vi "Update limits.vi"(8 "error in (no error)":errorcluster, 10 "Experiment.lvclass in":refnum<class "Experiment.lvclass">, 11 "Control-Client in":refnum<class "Control-Client.lvclass">) -> (0 "error out":errorcluster, 3 "Control-Client out":refnum<class "Control-Client.lvclass">)   [LabVIEW 2018, in "Control-Client.lvclass"]
uses:
  Control-Client.lvclass
  Experiments/Experiment.lvclass
  Control-Client.lvclass/Control-Client.ctl
  Experiments/Experiment.lvclass/Experiment.ctl
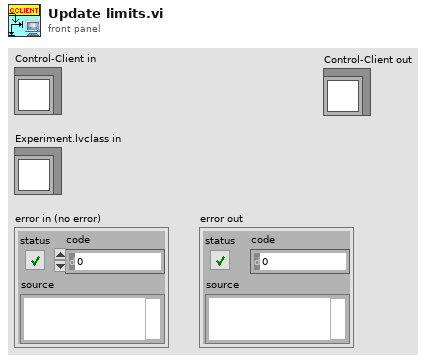
[diagram p1: front panel]
types:
  T1 = cluster{"From Time pix":i32, "To Time pix":i32, "From Wave pix":i32, "To Wave pix":i32}
  T2 = cluster{"waves slider":refnum<vi>, "times slider":refnum<vi>}
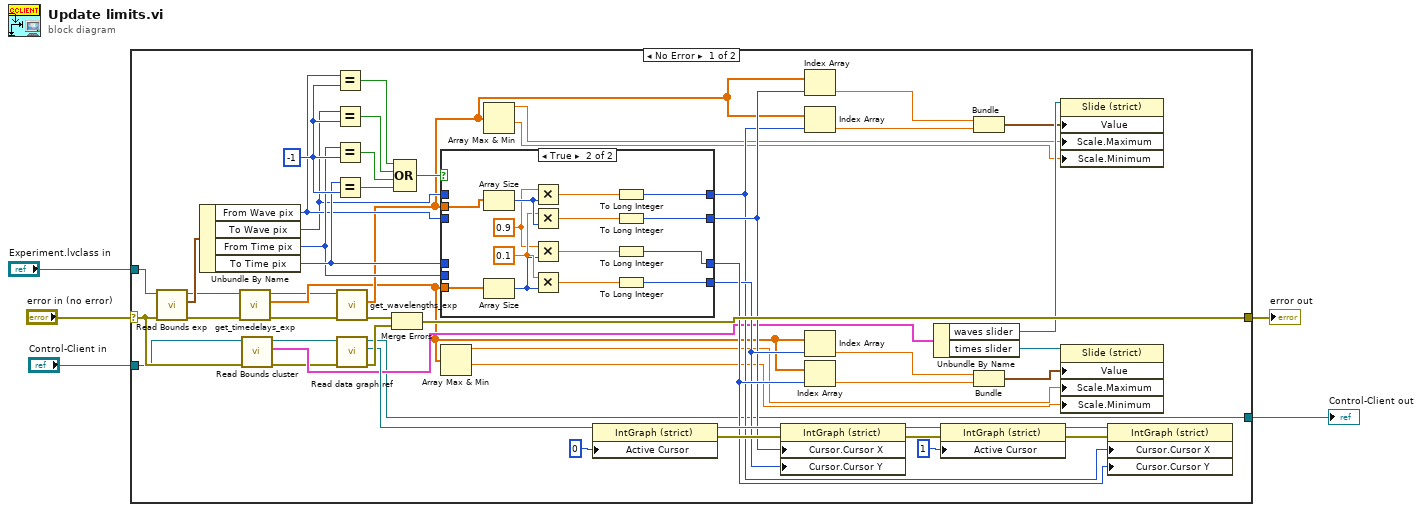
[diagram p0: block diagram]
diagram:
  n1 = case shown="No Error" "error in (no error)" {
    selector: "error in (no error)" -> [w43 w77]
    tunnel: "Experiment.lvclass in" -> [w57 _]
    tunnel: "Control-Client in" -> [w42 w76]
    tunnel: [w56 w77] -> w3
    tunnel: [w7 w76] -> w1
    frame No Error {
      w41 = -1 ("y")
      n2 = call "Read Bounds exp.vi"("error in (no error)"=w43, "Experiment in"=w57) -> ("error out"=w10:errorcluster, "Bounds pixels"=w44:T1, "Experiment out"=w12:refnum<class "Experiment.lvclass">)  [unwired: 7 in]
      n3 = Unbundle By Name(w44) -> ("From Wave pix"=w33:i32, "To Wave pix"=w29:i32, "From Time pix"=w34:i32, "To Time pix"=w35:i32)
      n4 = call "get_timedelays_exp.vi"("error in (no error)"=w10, "Experiment.lvclass in"=w12) -> ("error out"=w9:errorcluster, "timedelays"=w19:dbl[], "Experiment.lvclass out"=w11:refnum<class "Experiment.lvclass">)  [unwired: 7 in]
      n5 = call "Read Bounds cluster.vi"("error in (no error)"=w43, "Control-Client in"=w42) -> ("error out"=w6:errorcluster, "Bounds cluster"=w27:T2, "Control-Client out"=w8:refnum<class "Control-Client.lvclass">)  [unwired: 7 in]
      n6 = Equal?(x=w33, y=w41) -> (x = y?=w37:bool)
      n7 = Equal?(x=w29, y=w41) -> (x = y?=w38:bool)
      n8 = Equal?(x=w34, y=w41) -> (x = y?=w39:bool)
      n9 = Equal?(x=w35, y=w41) -> (x = y?=w40:bool)
      n10 = call "get_wavelengths_exp.vi"("error in (no error)"=w9, "Experiment.lvclass in"=w11) -> ("error out"=w45:errorcluster, "wavelengths"=w20:dbl[])  [unwired: 7 in, 1 out]
      n11 = call "Read data graph ref.vi"("error in (no error)"=w6, "Control-Client in"=w8) -> ("error out"=w55:errorcluster, "Exp data graph ref"=w54:refnum<vi>, "Control-Client out"=w7:refnum<class "Control-Client.lvclass">)  [unwired: 7 in]
      n12 = Merge Errors(w45, w55) -> (w56:errorcluster)
      n13 = Compound Arithmetic op=OR(w37, w38, w39, w40) -> (w31:bool)
      n14 = case shown="True" w31 {
        tunnel: [w61 w62] -> w36
        tunnel: w35 -> [w61 _]
        tunnel: [w60 w63] -> w32
        tunnel: w34 -> [w60 _]
        tunnel: [w59 w72] -> w30
        tunnel: w33 -> [w59 _]
        tunnel: [w58 w64] -> w28
        tunnel: w29 -> [w58 _]
        tunnel: w20 -> [_ w75]
        tunnel: w19 -> [_ w70]
        frame False {
        }
        frame True {
          w69 = 0.1 ("x")
          w68 = 0.9 ("x")
          n15 = Array Size(array=w75) -> (size(s)=w74:i32)
          n16 = Array Size(array=w70) -> (size(s)=w67:i32)
          n17 = Multiply(x=w68, y=w74) -> (x*y=w71:dbl)
          n18 = Multiply(x=w69, y=w74) -> (x*y=w73:dbl)
          n19 = Multiply(x=w68, y=w67) -> (x*y=w65:dbl)
          n20 = Multiply(x=w69, y=w67) -> (x*y=w66:dbl)
          n21 = To Long Integer(number=w71) -> (32bit integer=w64:i32)
          n22 = To Long Integer(number=w73) -> (32bit integer=w72:i32)
          n23 = To Long Integer(number=w65) -> (32bit integer=w62:i32)
          n24 = To Long Integer(number=w66) -> (32bit integer=w63:i32)
        }
      }
      n25 = Array Max & Min(array=w19) -> (max value=w16:dbl, min value=w15:dbl)  [unwired: 2 out]
      n26 = Array Max & Min(array=w20) -> (max value=w18:dbl, min value=w17:dbl)  [unwired: 2 out]
      n27 = property class="IntGraph (strict)"(reference=w54, "Active Cursor"=u32 0) -> (reference out=w52:refnum<vi>, error out=w51:errorcluster)  [unwired: 1 in]
      n28 = property class="IntGraph (strict)"(reference=w52, error in=w51, "Cursor.Cursor X"=w30, "Cursor.Cursor Y"=w32) -> (reference out=w50:refnum<vi>, error out=w49:errorcluster)
      n29 = Index Array(array=w20, index=w30) -> (element=w25:dbl)
      n30 = Index Array(array=w20, index=w28) -> (element=w24:dbl)
      n31 = Index Array(array=w19, index=w32) -> (element=w14:dbl)
      n32 = Index Array(array=w19, index=w36) -> (element=w13:dbl)
      n33 = Unbundle By Name(w27) -> ("waves slider"=w26:refnum<vi>, "times slider"=w22:refnum<vi>)
      n34 = property class="IntGraph (strict)"(reference=w50, error in=w49, "Active Cursor"=u32 1) -> (reference out=w48:refnum<vi>, error out=w47:errorcluster)
      n35 = Bundle("Numeric"=w25, "Numeric"=w24) -> (w23:cluster{"Numeric":dbl, "Numeric":dbl})  [unwired: 1 in]
      n36 = Bundle("delay"=w14, "delay"=w13) -> (w21:cluster{"delay":dbl, "delay":dbl})  [unwired: 1 in]
      n37 = property class="Slide (strict)"(reference=w26, "Value"=w23, "Scale.Maximum"=w18, "Scale.Minimum"=w17) -> ()  [unwired: 1 in, 2 out]
      n38 = property class="Slide (strict)"(reference=w22, "Value"=w21, "Scale.Maximum"=w16, "Scale.Minimum"=w15) -> ()  [unwired: 1 in, 2 out]
      n39 = property class="IntGraph (strict)"(reference=w48, error in=w47, "Cursor.Cursor X"=w28, "Cursor.Cursor Y"=w36) -> ()  [unwired: 2 out]
    }
    frame Error {
    }
  }
  "error out" <- w3
  "Control-Client out" <- w1
